vi "Example - Symbol Table.vi"(8 "Error In":errorcluster) -> (0 "Error Out":errorcluster)   [LabVIEW 2017, in "TwinCAT ADS.lvlib"]
uses:
  TwinCAT ADS.lvlib
  Low Level/TypeDefs/AMS.ctl
  High Level/PLC/PLC.lvlib
panel:
  in  "Router":string="127.0.0.1"
  in  "AMS":T1={"Target Net ID"="127.0.0.1.1.1", "Target Port"=851, "Source Net ID"="127.0.0.1.1.1", "Source Port"=10000}
  out "Table":string[][](table)
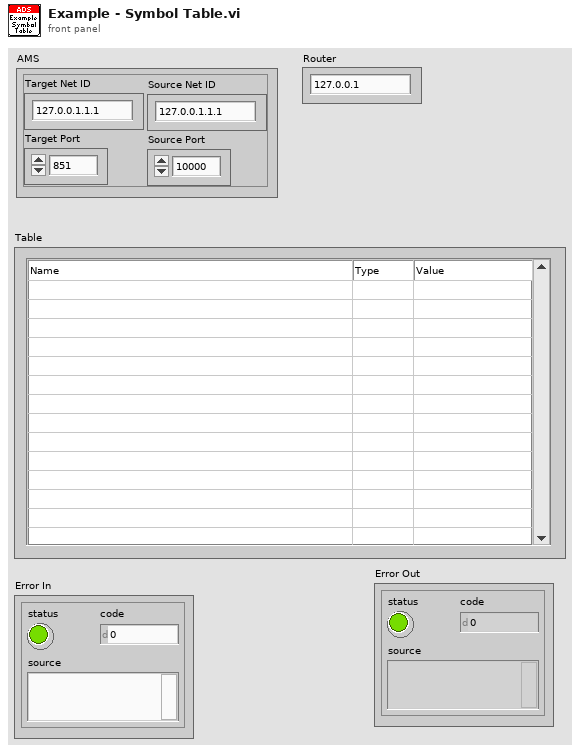
[diagram p1: front panel]
types:
  T1 = typedef "TwinCAT ADS.lvlib/AMS.ctl" = cluster{"Target Net ID":string, "Target Port":u16, "Source Net ID":string, "Source Port":u16}
  T2 = typedef "TwinCAT ADS.lvlib/AMS Connection.ctl" = cluster{"AMS":T1, "Timeout":i32, "TCP Connection Ref":refnum<k5>}
  T3 = typedef "TwinCAT ADS.lvlib/PLC.lvlib/AdsSymbolEntry.ctl" = cluster{"entryLength":i32, "iGroup":i32, "iOffs":i32, "size":i32, "dataType":T4, "flags":i32, "nameLength":i16, "typeLength":i16, "commentLength":i16, "Name":string, "Type":string, "Comment":string}
  T4 = typedef "dataType.ctl" = u16
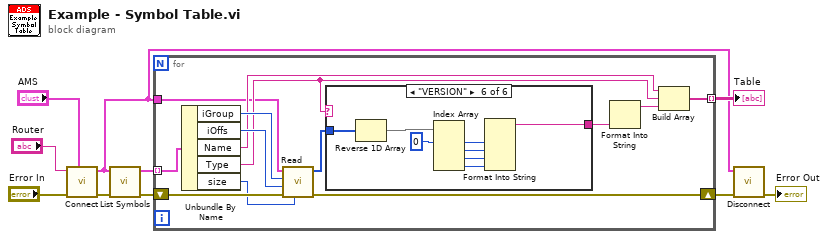
[diagram p0: block diagram]
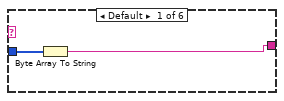
[diagram p2: hidden frame]
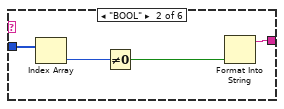
[diagram p3: hidden frame]
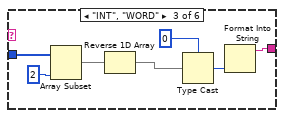
[diagram p4: hidden frame]
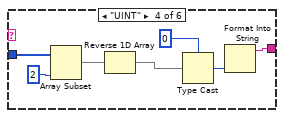
[diagram p5: hidden frame]
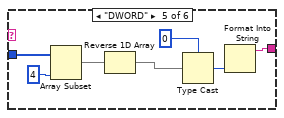
[diagram p6: hidden frame]
diagram:
  n1 = call "Connect.vi"("AMS"="AMS", "Error In"="Error In", "Router"="Router") -> ("Error Out"=w6:errorcluster, "AMS Connection"=w1:T2)  [unwired: 5 in, 2 out]
  n2 = call "List Symbols.vi"("error in (no error)"=w6, "AMS Connection In"=w1) -> ("Error Out"=w5:errorcluster, "Symbols"=w2:T3[])  [unwired: 8 in]
  n3 = for {
    tunnel: w2 -> [w23] mode=indexing
    shift-right: [w19] -> w4
    shift-left: w5 -> [w20]
    tunnel: [w16] -> w3 mode=indexing
    tunnel: w1 -> [w12]
    n4 = Unbundle By Name(w23) -> ("iGroup"=w22:i32, "iOffs"=w21:i32, "Name"=w18:string, "Type"=w15:string, "size"=w13:i32)
    n5 = call "Read.vi"("Read Length"=w13, "Error In"=w20, "Offset"=w21, "Index Group"=w22, "AMS Connection In"=w12) -> ("Error Out"=w19:errorcluster, "Data"=w11:u8[])  [unwired: 4 in, 1 out]
    n6 = case shown="\"VERSION\"" w15 {
      tunnel: [w24 w26 w35 w42 w49 w58] -> w14
      tunnel: w11 -> [w25 w29 w36 w43 w50 w56]
      frame Default {
        n7 = Byte Array To String(unsigned byte array=w25) -> (string=w24:string)
      }
      frame "BOOL" {
        n8 = Index Array(array=w29) -> (element=w28:u8)  [unwired: 1 in]
        n9 = Not Equal To 0?(x=w28) -> (x != 0?=w27:bool)
        n10 = Format Into String(w27) -> (resulting string=w26:string)  [unwired: 3 in, 1 out]
      }
      frame "INT", "WORD" {
        n11 = Array Subset(array=w36, length=2) -> (w33:u8[])  [unwired: 1 in]
        n12 = Reverse 1D Array(array=w33) -> (reversed array=w30:u8[])
        n13 = Type Cast(type=i16 0 ("length"), x=w30) -> (*(type *) &x=w31:i16)
        n14 = Format Into String(w31) -> (resulting string=w35:string)  [unwired: 3 in, 1 out]
      }
      frame "UINT" {
        n15 = Array Subset(array=w43, length=2) -> (w40:u8[])  [unwired: 1 in]
        n16 = Reverse 1D Array(array=w40) -> (reversed array=w37:u8[])
        n17 = Type Cast(type=u16 0 ("length"), x=w37) -> (*(type *) &x=w38:u16)
        n18 = Format Into String(w38) -> (resulting string=w42:string)  [unwired: 3 in, 1 out]
      }
      frame "DWORD" {
        n19 = Array Subset(array=w50, length=4) -> (w47:u8[])  [unwired: 1 in]
        n20 = Reverse 1D Array(array=w47) -> (reversed array=w44:u8[])
        n21 = Type Cast(type=i64 0 ("length"), x=w44) -> (*(type *) &x=w45:i64)
        n22 = Format Into String(w45) -> (resulting string=w49:string)  [unwired: 3 in, 1 out]
      }
      frame "VERSION" {
        n23 = Reverse 1D Array(array=w56) -> (reversed array=w51:u8[])
        n24 = Index Array(array=w51, index #1=0 ("index")) -> (element #1=w55:u8, element #2=w54:u8, element #3=w53:u8, element #4=w52:u8)  [unwired: 3 in]
        n25 = Format Into String(w55, w54, w53, w52) -> (resulting string=w58:string)  [unwired: 3 in, 1 out]
      }
    }
    n26 = Format Into String(w14) -> (resulting string=w17:string)  [unwired: 3 in, 1 out]
    n27 = Build Array(w18, w15, w17) -> (w16:string[])
  }
  "Table" <- w3
  n28 = call "Disconnect.vi"("Error In"=w4, "AMS Connection"=w1) -> ("Error Out"=→"Error Out":errorcluster)  [unwired: 9 in]
